vi "Storage Immediate.vi"(9 "Transfer Speed":dbl, 10 "Spindexer Speed":dbl, 11 "Operation":T1) -> ()   [LabVIEW 2019]
uses:
  <vilib>/Rock Robotics/WPI/Framework/Command Status Info.ctl
  <vilib>/Rock Robotics/WPI/Framework/Completion Status.ctl
  <vilib>/Rock Robotics/WPI/Framework/Completion Notifier.ctl
  Implementation/Storage Operations.ctl
  Implementation/Storage Setpoints.ctl
panel:
  in  "Description":string
  out "Command Info Out":T2
  in  "Command Info In":T2
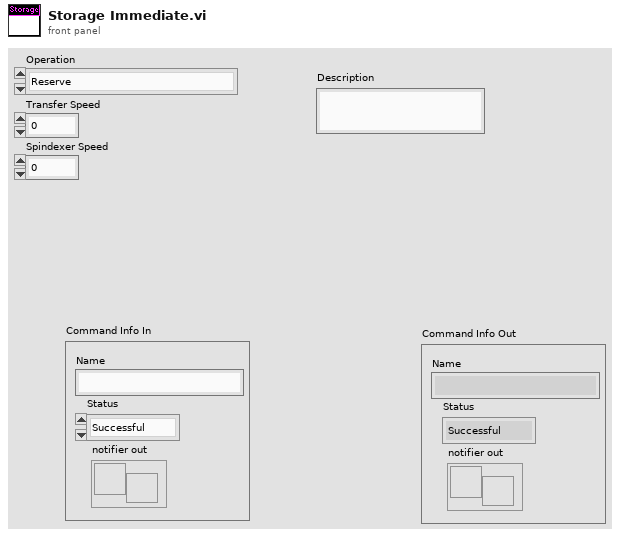
[diagram p1: front panel]
types:
  T1 = typedef "Storage Operations.ctl" = enum16{"Reserve", "Read Current", "Immediate", "Intake", "Shoot", "Override"}
  T2 = typedef "Command Status Info.ctl" = cluster{"Name":string, "Status":T3, "notifier out":T4}
  T3 = typedef "Completion Status.ctl" = enum16{"Successful", "Aborted", "Incomplete"}
  T4 = typedef "Completion Notifier.ctl" = refnum<notifier>
  T5 = typedef "Storage Setpoints.ctl" = cluster{"Operation":T1, "Transfer Speed":dbl, "Spindexer Speed":dbl}
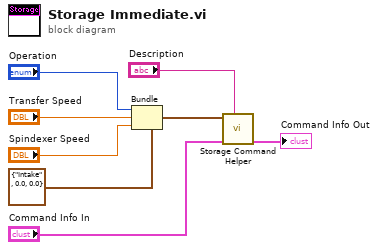
[diagram p0: block diagram]
diagram:
  n1 = Bundle(cluster=T5 {"Operation"=enum."Intake", "Transfer Speed"=0.0, "Spindexer Speed"=0.0} ("SubSystem Data"), "Operation"="Operation", "Transfer Speed"="Transfer Speed", "Spindexer Speed"="Spindexer Speed") -> (w4:T5)
  n2 = call "Storage Command Helper.vi"("Description"="Description", "Command Info In"="Command Info In", "SubSystem Data"=w4) -> ("Command Info Out"=→"Command Info Out":T2)  [unwired: 6 in, 2 out]
